vi "avaerage_attempt.vi"() -> ()   [LabVIEW 2020]
panel:
  in  "Stop Button":bool
  in  "Save data":bool
  in  "File_name":path=path "saved_data"
  out "XY Graph":cluster{"Y":dbl[], "Y":dbl[]}[](graph)
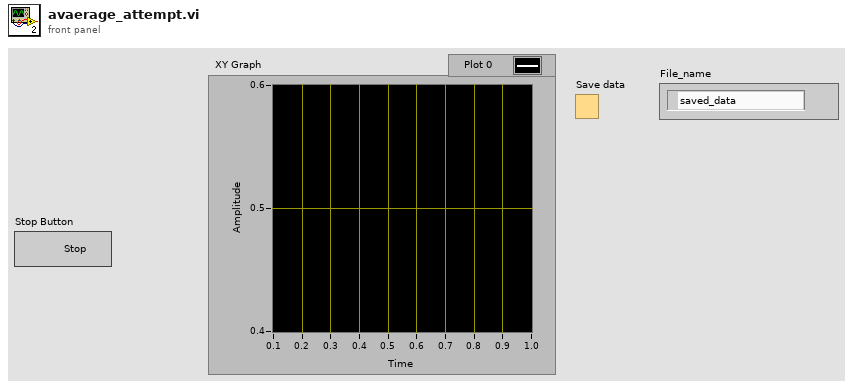
[diagram p1: front panel]
types:
  T1 = enum16{"open", "replace", "create", "open or create", "replace or create", "replace or create with confirmation"}
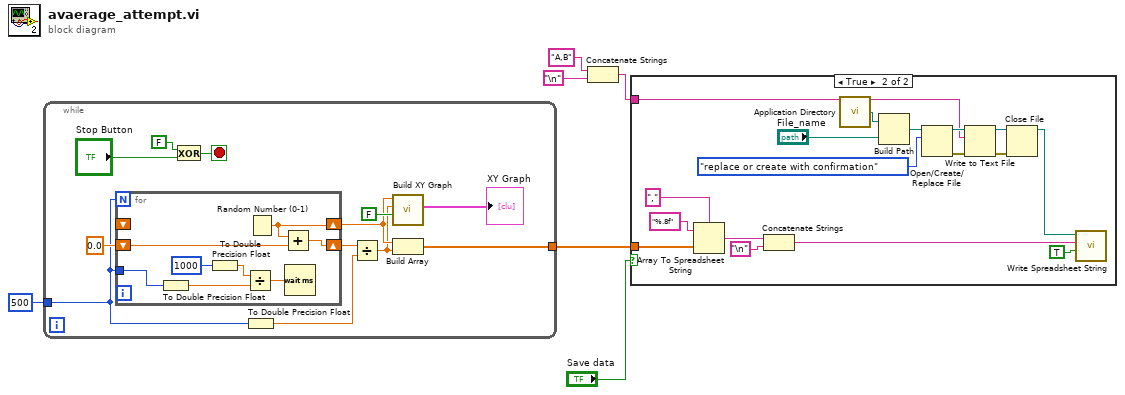
[diagram p0: block diagram]
diagram:
  n1 = while {
    tunnel: 500 -> [w15]
    tunnel: [w10] -> w4
    stop <- w9 stop-if-true
    n2 = for {
      N: w15 -> [_]
      tunnel: w15 -> [w22]
      shift-right: [w24] -> w17
      shift-left: 0.0 -> [w25]
      shift-right: [w19] -> w12
      shift-left: _ -> [_]
      n3 = To Double Precision Float(number=w22) -> (double precision float=w20:dbl)
      n4 = To Double Precision Float(number=u32 1000 ("milliseconds to wait")) -> (double precision float=w21:dbl)
      n5 = Divide(x=w21, y=w20) -> (x/y=w26:dbl)
      n6 = Random Number (0-1)() -> (number: 0 to 1=w19:dbl)
      n7 = Add(x=w19, y=w25) -> (x+y=w24:dbl)
      n8 = Wait (ms)(milliseconds to wait=w26) -> ()  [unwired: 1 out]
    }
    n9 = Exclusive Or(1:"Stop Button", 2:FALSE) -> (0:w9:bool)
    n10 = To Double Precision Float(number=w15) -> (double precision float=w16:dbl)
    n11 = Divide(x=w17, y=w16) -> (x/y=w11:dbl)
    n12 = call "Build XY Graph"("Reset"=FALSE, "Y Input"=w11, "X Input"=w12) -> ("XY Graph"=→"XY Graph":cluster{"X":dbl[], "Y":dbl[]}[])  [unwired: 7 in, 1 out]
    n13 = Build Array(w12, w11) -> (w10:dbl[])
  }
  n14 = Concatenate Strings("A,B", "\n") -> (w2:string)
  n15 = case shown="True" "Save data" {
    tunnel: w2 -> [_ w31]
    tunnel: w4 -> [_ w30]
    frame False {
    }
    frame True {
      n16 = Array To Spreadsheet String(delimiter (Tab)=",", array=w30, 3:"%.8f" ("format string")) -> (spreadsheet string=w29:string)
      n17 = Concatenate Strings(w29, "\n") -> (w27:string)
      n18 = call <vilib>:"Application Directory.vi"() -> ("Application Directory"=w41:path)
      n19 = Build Path(base path=w41, name or relative path="File_name") -> (appended path=w39:path)
      n20 = Open/Create/Replace File(file path (use dialog)=w39, operation (0:open)=T1."replace or create with confirmation") -> (refnum out=w35:refnum<file>, error out=w34:errorcluster)  [unwired: 4 in, 1 out]
      n21 = Write to Text File(file (use dialog)=w35, text=w31, error in=w34) -> (refnum out=w33:refnum<file>, error out=w32:errorcluster)  [unwired: 1 in, 1 out]
      n22 = Close File(refnum=w33, error in=w32) -> (path=w38:path)  [unwired: 1 out]
      n23 = call <vilib>:"Write Spreadsheet String.vi"("append to file? (new file:F)"=TRUE, "spreadsheet string"=w27, "file path (dialog if empty)"=w38) -> ()  [unwired: 7 in, 2 out]
    }
  }
